vi "Haar小波基矢.vi"() -> ()   [LabVIEW 2016]
uses:
  <vilib>/Analysis/Matrix/Numeric/Conversions/Array To Matrix - RA2.vi
  <vilib>/Analysis/Matrix/Numeric/Multiply/Multiply - RM,RM.vi
  <vilib>/Analysis/Matrix/Numeric/Conversions/Matrix To Array - RM.vi
  <vilib>/Analysis/Matrix/NI_Matrix.lvlib
panel:
  out "Numeric":i32
  out "show":dbl[][](graph)
  in  "path to JPEG file":path
  out "read":u32[][](graph)
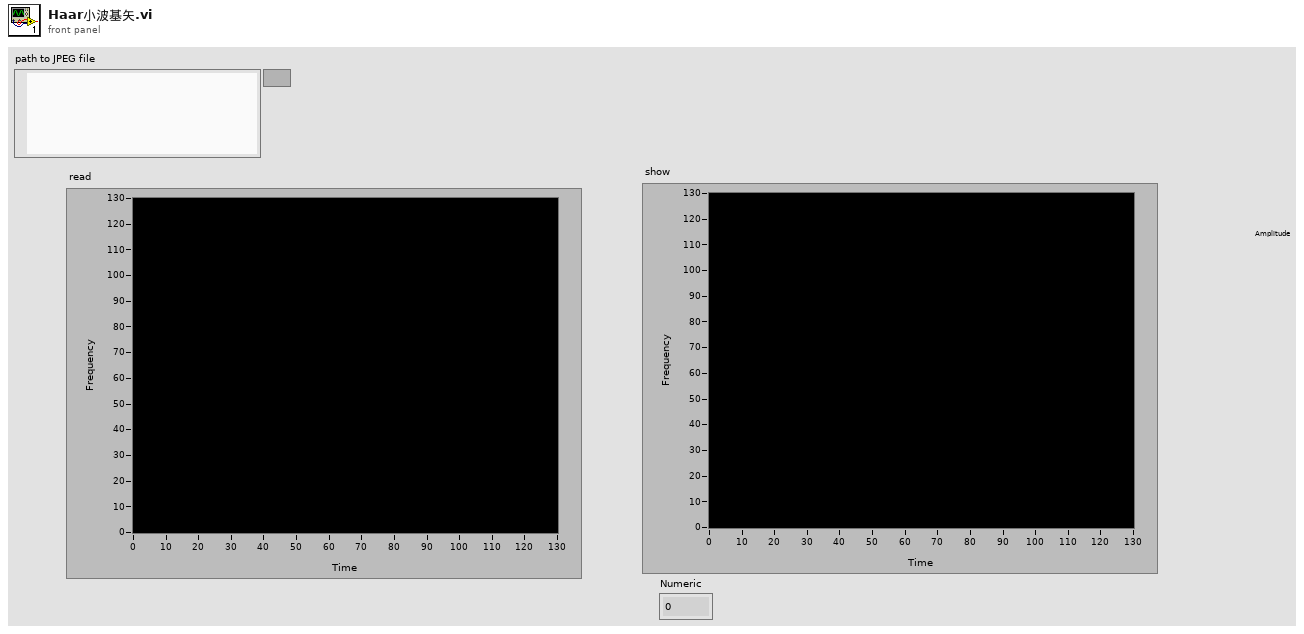
[diagram p1: front panel]
types:
  T1 = typedef "imagedata.ctl" = cluster{"image type":i32, "image depth":i32, "image":u8[], "mask":u8[], "colors":u32[], "Rectangle":cluster{"left":i16, "top":i16, "right":i16, "bottom":i16}}
  T2 = typedef "NI_Matrix.lvlib/RealMatrix.ctl" = dbl[][]
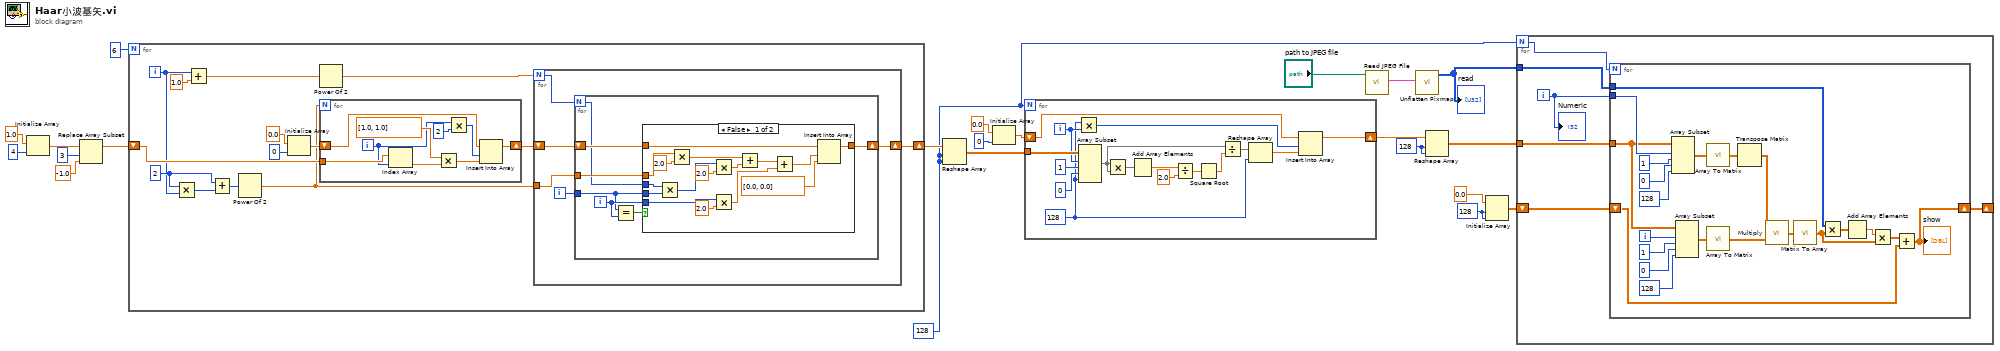
[diagram p0: block diagram]
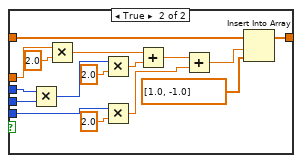
[diagram p2: hidden frame]
diagram:
  w2 = 128 ("dimension size")
  w13 = 128 ("dimension size")
  w6 = 128 ("dimension size")
  n1 = Initialize Array(1.0 ("element"), 4 ("dimension size")) -> (w20:dbl[])
  n2 = Replace Array Subset(array=w20, new element=-1.0 ("new element/subarray"), index=3) -> (w16:dbl[])
  n3 = for {
    N: 6 -> [_]
    shift-right: [w24] -> w15
    shift-left: w16 -> [w30]
    i -> [w27]
    w35 = 2 ("x")
    n4 = Multiply(x=w35, y=w27) -> (x*y=w34:i32)
    n5 = Add(x=w27, y=1.0) -> (x+y=w29:dbl)
    n6 = Add(x=w35, y=w34) -> (x+y=w36:i32)
    n7 = Power Of 2(x=w36) -> (2^x=w25:dbl)
    n8 = Initialize Array(0.0 ("element"), 0 ("dimension size")) -> (w31:dbl[])
    n9 = Power Of 2(x=w29) -> (2^x=w23:dbl)
    n10 = for {
      N: w25 -> [_]
      tunnel: w30 -> [w89]
      shift-right: [w81] -> w26
      shift-left: w31 -> [w88]
      i -> [w84]
      n11 = Index Array(array=w89, index=w84) -> (element=w85:dbl)
      n12 = Multiply(x=dbl[] [1.0, 1.0] ("array"), y=w85) -> (x*y=w87:dbl[])
      n13 = Multiply(x=w84, y=2 ("x")) -> (x*y=w82:i32)
      n14 = Insert Into Array(array=w88, index=w82, new element=w87) -> (w81:dbl[])
    }
    n15 = for {
      N: w23 -> [w41]
      shift-right: [w39] -> w24
      shift-left: w26 -> [w40]
      tunnel: w25 -> [w38]
      i -> [w37]
      n16 = for {
        N: w41 -> [w45]
        shift-right: [w42] -> w39
        shift-left: w40 -> [w47]
        tunnel: w37 -> [w43]
        tunnel: w38 -> [w46]
        i -> [w44]
        n17 = Equal?(x=w43, y=w44) -> (x = y?=w48:bool)
        n18 = case shown="False" w48 {
          tunnel: w47 -> [w64 w67]
          tunnel: w46 -> [w61 w71]
          tunnel: w45 -> [w59 w70]
          tunnel: w43 -> [w58 w69]
          tunnel: w44 -> [w51 w68]
          tunnel: [w50 w66] -> w42
          frame False {
            n19 = Multiply(x=w59, y=w58) -> (x*y=w54:i32)
            n20 = Multiply(x=w61, y=2.0) -> (x*y=w60:dbl)
            n21 = Multiply(x=w54, y=2.0) -> (x*y=w55:dbl)
            n22 = Multiply(x=w51, y=2.0) -> (x*y=w52:dbl)
            n23 = Add(x=w60, y=w55) -> (x+y=w57:dbl)
            n24 = Add(x=w57, y=w52) -> (x+y=w49:dbl)
            n25 = Insert Into Array(array=w64, index=w49, new element=dbl[] [0.0, 0.0] ("array")) -> (w50:dbl[])
          }
          frame True {
            n26 = Multiply(x=w70, y=w69) -> (x*y=w75:i32)
            n27 = Multiply(x=w71, y=2.0) -> (x*y=w79:dbl)
            n28 = Multiply(x=w75, y=2.0) -> (x*y=w76:dbl)
            n29 = Multiply(x=w68, y=2.0) -> (x*y=w73:dbl)
            n30 = Add(x=w79, y=w76) -> (x+y=w78:dbl)
            n31 = Add(x=w78, y=w73) -> (x+y=w72:dbl)
            n32 = Insert Into Array(array=w67, index=w72, new element=dbl[] [1.0, -1.0] ("array")) -> (w66:dbl[])
          }
        }
      }
    }
  }
  n33 = Reshape Array(w15, w6, w6) -> (w4:dbl[][])
  n34 = Initialize Array(0.0 ("element"), 0 ("dimension size")) -> (w5:dbl[])
  n35 = for {
    N: w6 -> [_]
    shift-right: [w93] -> w3
    shift-left: w5 -> [w95]
    tunnel: w4 -> [w105]
    i -> [w96]
    w91 = 128 ("length")
    n36 = Multiply(x=w91, y=w96) -> (x*y=w94:i32)
    n37 = Array Subset(array=w105, index (row)=w96, length (row)=1 ("length"), index (col)=0 ("index"), length (col)=w91) -> (w102:dbl[][])
    n38 = Multiply(x=w102, y=w102) -> (x*y=w100:dbl[][])
    n39 = Add Array Elements(numeric array=w100) -> (sum=w99:dbl)
    n40 = Divide(x=w99, y=2.0) -> (x/y=w97:dbl)
    n41 = Square Root(x=w97) -> (sqrt(x)=w101:dbl)
    n42 = Divide(x=w102, y=w101) -> (x/y=w92:dbl[][])
    n43 = Reshape Array(w92, w91) -> (w90:dbl[])
    n44 = Insert Into Array(array=w95, index=w94, new element=w90) -> (w93:dbl[])
  }
  n45 = call <vilib>:"Read JPEG File.vi"("path to JPEG file"="path to JPEG file") -> ("image data"=w11:T1)  [unwired: 8 in, 2 out]
  n46 = call <vilib>:"Unflatten Pixmap.vi"("image data"=w11) -> ("24-bit pixmap"=w14:u32[][])  [unwired: 4 in, 6 out]
  "read" <- w14
  n47 = Reshape Array(w3, w2, w2) -> (w1:dbl[][])
  n48 = Initialize Array(0.0 ("element"), w13, w13) -> (w9:dbl[][])
  n49 = for {
    N: w6 -> [w111]
    tunnel: w1 -> [w110]
    tunnel: w14 -> [w108]
    shift-right: [w106] -> _
    shift-left: w9 -> [w107]
    i -> [w109]
    n50 = for {
      N: w111 -> [_]
      tunnel: w110 -> [w126]
      tunnel: w109 -> [w133]
      tunnel: w108 -> [w122]
      shift-right: [w113] -> w106
      shift-left: w107 -> [w118]
      i -> [w125]
      n51 = Array Subset(array=w126, index (row)=w133, length (row)=1 ("length"), index (col)=0 ("index"), length (col)=128 ("length")) -> (w124:dbl[][])
      n52 = Array Subset(array=w126, index (row)=w125, length (row)=1 ("length"), index (col)=0 ("index"), length (col)=128 ("length")) -> (w123:dbl[][])
      n53 = call-poly <vilib>:"Array To Matrix.vi"("Real 2D Array"=w124) -> ("Real Matrix"=w116:T2)
      n54 = call-poly <vilib>:"Array To Matrix.vi"("Real 2D Array"=w123) -> ("Real Matrix"=w117:T2)
      n55 = Transpose Matrix(1:w116) -> (0:w115:T2)
      n56 = call-poly <vilib>:"Multiply.vi"("Real Matrix B"=w117, "Real Matrix A"=w115) -> ("A * B"=w114:T2)
      n57 = call-poly <vilib>:"Matrix To Array.vi"("Real Matrix"=w114) -> ("Real 2D Array"=w112:dbl[][])
      n58 = Multiply(x=w122, y=w112) -> (x*y=w121:dbl[][])
      n59 = Add Array Elements(numeric array=w121) -> (sum=w120:dbl)
      n60 = Multiply(x=w120, y=w112) -> (x*y=w119:dbl[][])
      n61 = Add(x=w119, y=w118) -> (x+y=w113:dbl[][])
      "show" <- w113
    }
    "Numeric" <- w109
  }
